vi "KHE - Load Settings.vi"(8 "error in (no error)":errorcluster) -> (0 "error out":errorcluster, 1 "Instrument Locations":T7, 2 "Instruments":T6={"Magnet"=enum."Manual", "Ammeter"=enum."648X", "Current Source"=enum."622X", "Switch"=enum."3706A", "Voltmeter"=enum."2182A"})   [LabVIEW 2016]
uses:
  Hall Effect Library/Public/Controls/Magnets.ctl
  Hall Effect Library/Public/Controls/Ammeters.ctl
  Hall Effect Library/Public/Controls/I-Sources.ctl
  Hall Effect Library/Public/Controls/Switches.ctl
  Hall Effect Library/Public/Controls/Voltmeters.ctl
  Hall Effect Library/Hall Effect Library.lvlib
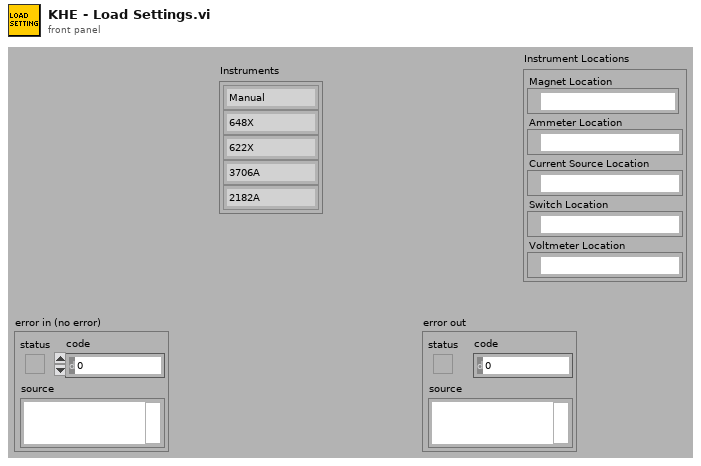
[diagram p1: front panel]
types:
  T1 = typedef "Hall Effect Library.lvlib/Magnets.ctl" = enum16{"Manual"}
  T2 = typedef "Hall Effect Library.lvlib/Ammeters.ctl" = enum16{"None", "648X"}
  T3 = typedef "Hall Effect Library.lvlib/I-Sources.ctl" = enum16{"622X", "26XX"}
  T4 = typedef "Hall Effect Library.lvlib/Switches.ctl" = enum16{"3706A"}
  T5 = typedef "Hall Effect Library.lvlib/Voltmeters.ctl" = enum16{"2000", "2182A", "3706A"}
  T6 = cluster{"Magnet":T1, "Ammeter":T2, "Current Source":T3, "Switch":T4, "Voltmeter":T5}
  T7 = cluster{"Magnet Location":refnum<visa-resource-name>, "Ammeter Location":refnum<visa-resource-name>, "Current Source Location":refnum<visa-resource-name>, "Switch Location":refnum<visa-resource-name>, "Voltmeter Location":refnum<visa-resource-name>}
  T8 = cluster{"Instruments":cluster{"Magnet":T1, "Ammeter":T2, "Current Source":T3, "Switch":T4, "Voltmeter":T5}, "Instrument Locations":cluster{"Magnet Location":refnum<visa-resource-name>, "Ammeter Location":refnum<visa-resource-name>, "Current Source Location":refnum<visa-resource-name>, "Switch Location":refnum<visa-resource-name>, "Voltmeter Location":refnum<visa-resource-name>}}
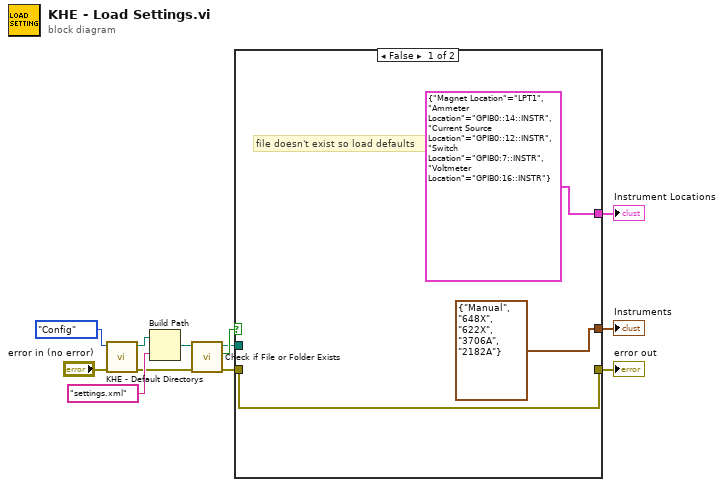
[diagram p0: block diagram]
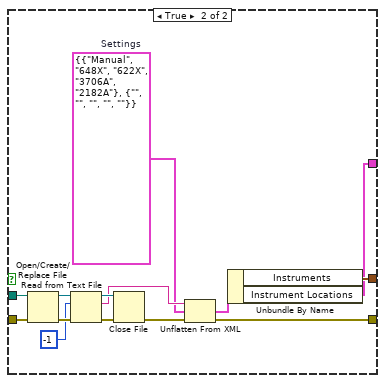
[diagram p2: hidden frame]
diagram:
  n1 = call "KHE - Default Directorys.vi"("error in (no error)"="error in (no error)", "Directory"=enum16{"Root", "Config", "Results"}."Config") -> ("error out"=w3:errorcluster, "Path Out"=w4:path)  [unwired: 8 out]
  n2 = Build Path(base path=w4, name or relative path="settings.xml") -> (appended path=w11:path)
  n3 = call <vilib>:"Check if File or Folder Exists.vi"("error in (no error)"=w3, "path"=w11) -> ("error out"=w8:errorcluster, "file or folder exists?"=w10:bool, "dup path"=w9:path)  [unwired: 7 out]
  n4 = case shown="False" w10 {
    tunnel: w9 -> [_ w28]
    tunnel: w8 -> [w15 w29]
    tunnel: [T6 {"Magnet"=enum."Manual", "Ammeter"=enum."648X", "Current Source"=enum."622X", "Switch"=enum."3706A", "Voltmeter"=enum."2182A"} ("Instruments") w18] -> w7
    tunnel: [T7 {"Magnet Location"="LPT1", "Ammeter Location"="GPIB0::14::INSTR", "Current Source Location"="GPIB0::12::INSTR", "Switch Location"="GPIB0:7::INSTR", "Voltmeter Location"="GPIB0:16::INSTR"} ("Instrument Locations") w17] -> w6
    tunnel: [w15 w16] -> w5
    frame False {
      # "file doesn't exist so load defaults"
    }
    frame True {
      w20 = T8 {"Instruments"={"Magnet"=enum."Manual", "Ammeter"=enum."648X", "Current Source"=enum."622X", "Switch"=enum."3706A", "Voltmeter"=enum."2182A"}, "Instrument Locations"={"Magnet Location"="", "Ammeter Location"="", "Current Source Location"="", "Switch Location"="", "Voltmeter Location"=""}}  # Settings
      n5 = Open/Create/Replace File(file path (use dialog)=w28, error in=w29) -> (refnum out=w24:refnum<file>, error out=w27:errorcluster)  [unwired: 5 out]
      n6 = Read from Text File(file (use dialog)=w24, count=-1, error in=w27) -> (refnum out=w25:refnum<file>, text=w22:string, error out=w26:errorcluster)  [unwired: 2 out]
      n7 = Close File(refnum=w25, error in=w26) -> (error out=w21:errorcluster)  [unwired: 1 out]
      n8 = Unflatten From XML(xml string=w22, type=w20, error in (no error)=w21) -> (value=w19:T8, error out=w16:errorcluster)
      n9 = Unbundle By Name(w19) -> ("Instruments"=w18:T6, "Instrument Locations"=w17:T7)
    }
  }
  "Instruments" <- w7
  "Instrument Locations" <- w6
  "error out" <- w5
